vi "Calculate sensor threshold.vi"(0 "设置的起搏幅度":dbl=4.0, 5 "设定脉宽":dbl, 7 "Test Result":waveform(dbl), 9 "波形图":waveform(dbl)[](array[waveform])=[{"t0"=timestamp(3440194019.9959836 s since 1904-01-01), "dt"=1.9999999999999944e-06, "Y"=array[49999 elements], "attributes"=variant("NI_ChannelName"=variant(string "6259A/ai15"), "NI_UnitDescription"=variant(string "Volts"))}, {"t0"=timestamp(3440194019.9959836 s since 1904-01-01), "dt"=1.9999999999999944e-06, "Y"=array[49999 elements], "attributes"=variant("NI_ChannelName"=variant(string "6259A/ai21"), "NI_UnitDescription"=variant(string "Volts"))}]) -> (2 "LE":dbl, 3 "TE":dbl, 4 "VP max":dbl, 6 "VP （200u（起搏幅度））":dbl, 8 "pluse width":dbl, 10 "Vpgb（起搏幅度） 国标1":dbl, 11 "Waveform Graph Cal":waveform(dbl)(graph), 12 "VP/vh":dbl, 14 "Vpgb/vh":dbl, 15 "PW":dbl)   [LabVIEW 2016]
panel:
  out "b":dbl
  out "k":dbl
  out "element":dbl
  out "dt":dbl
  out "Waveform Graph":waveform(dbl)(graph)
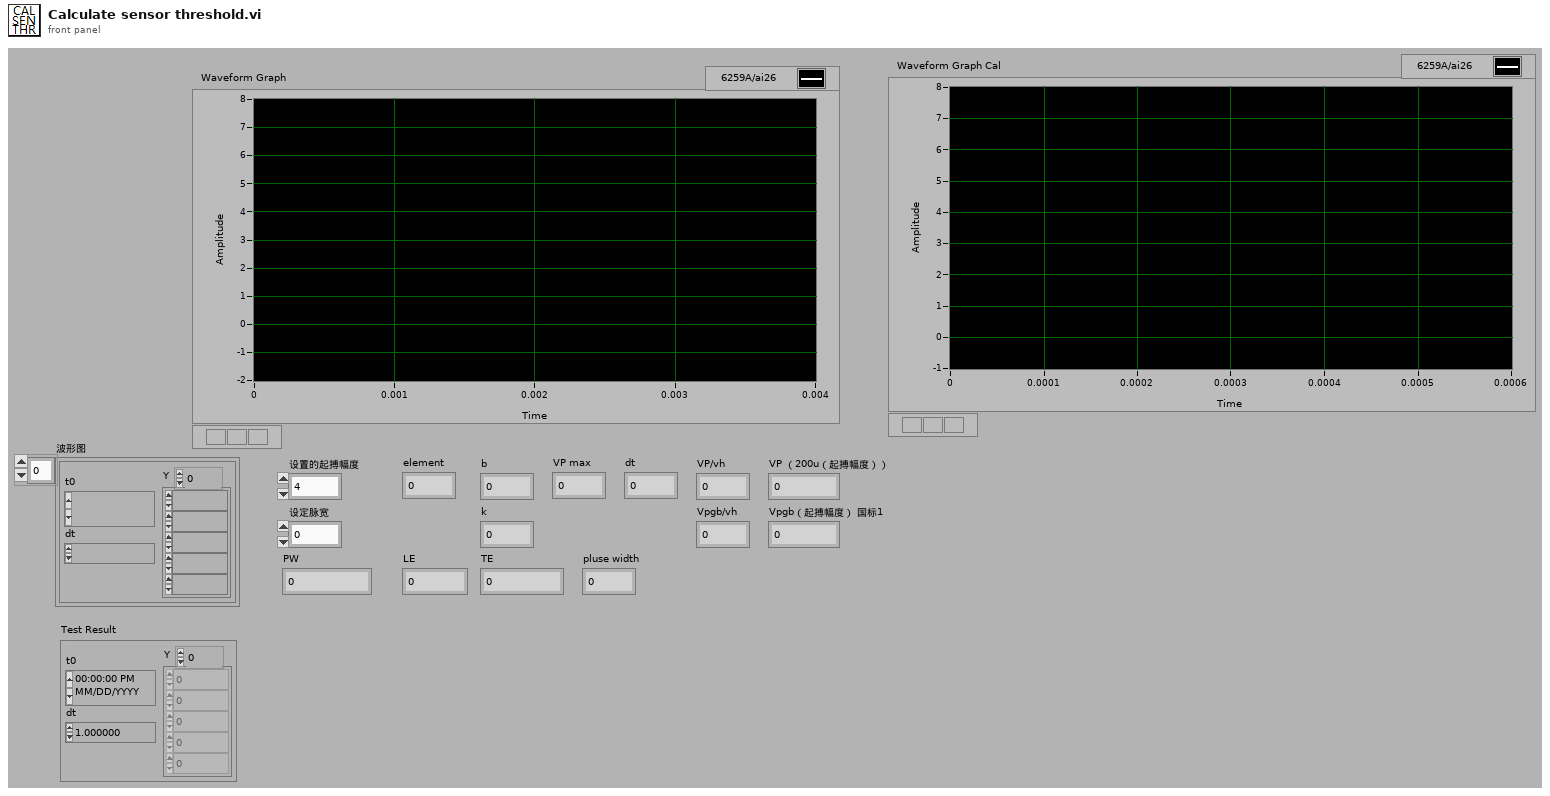
[diagram p1: front panel]
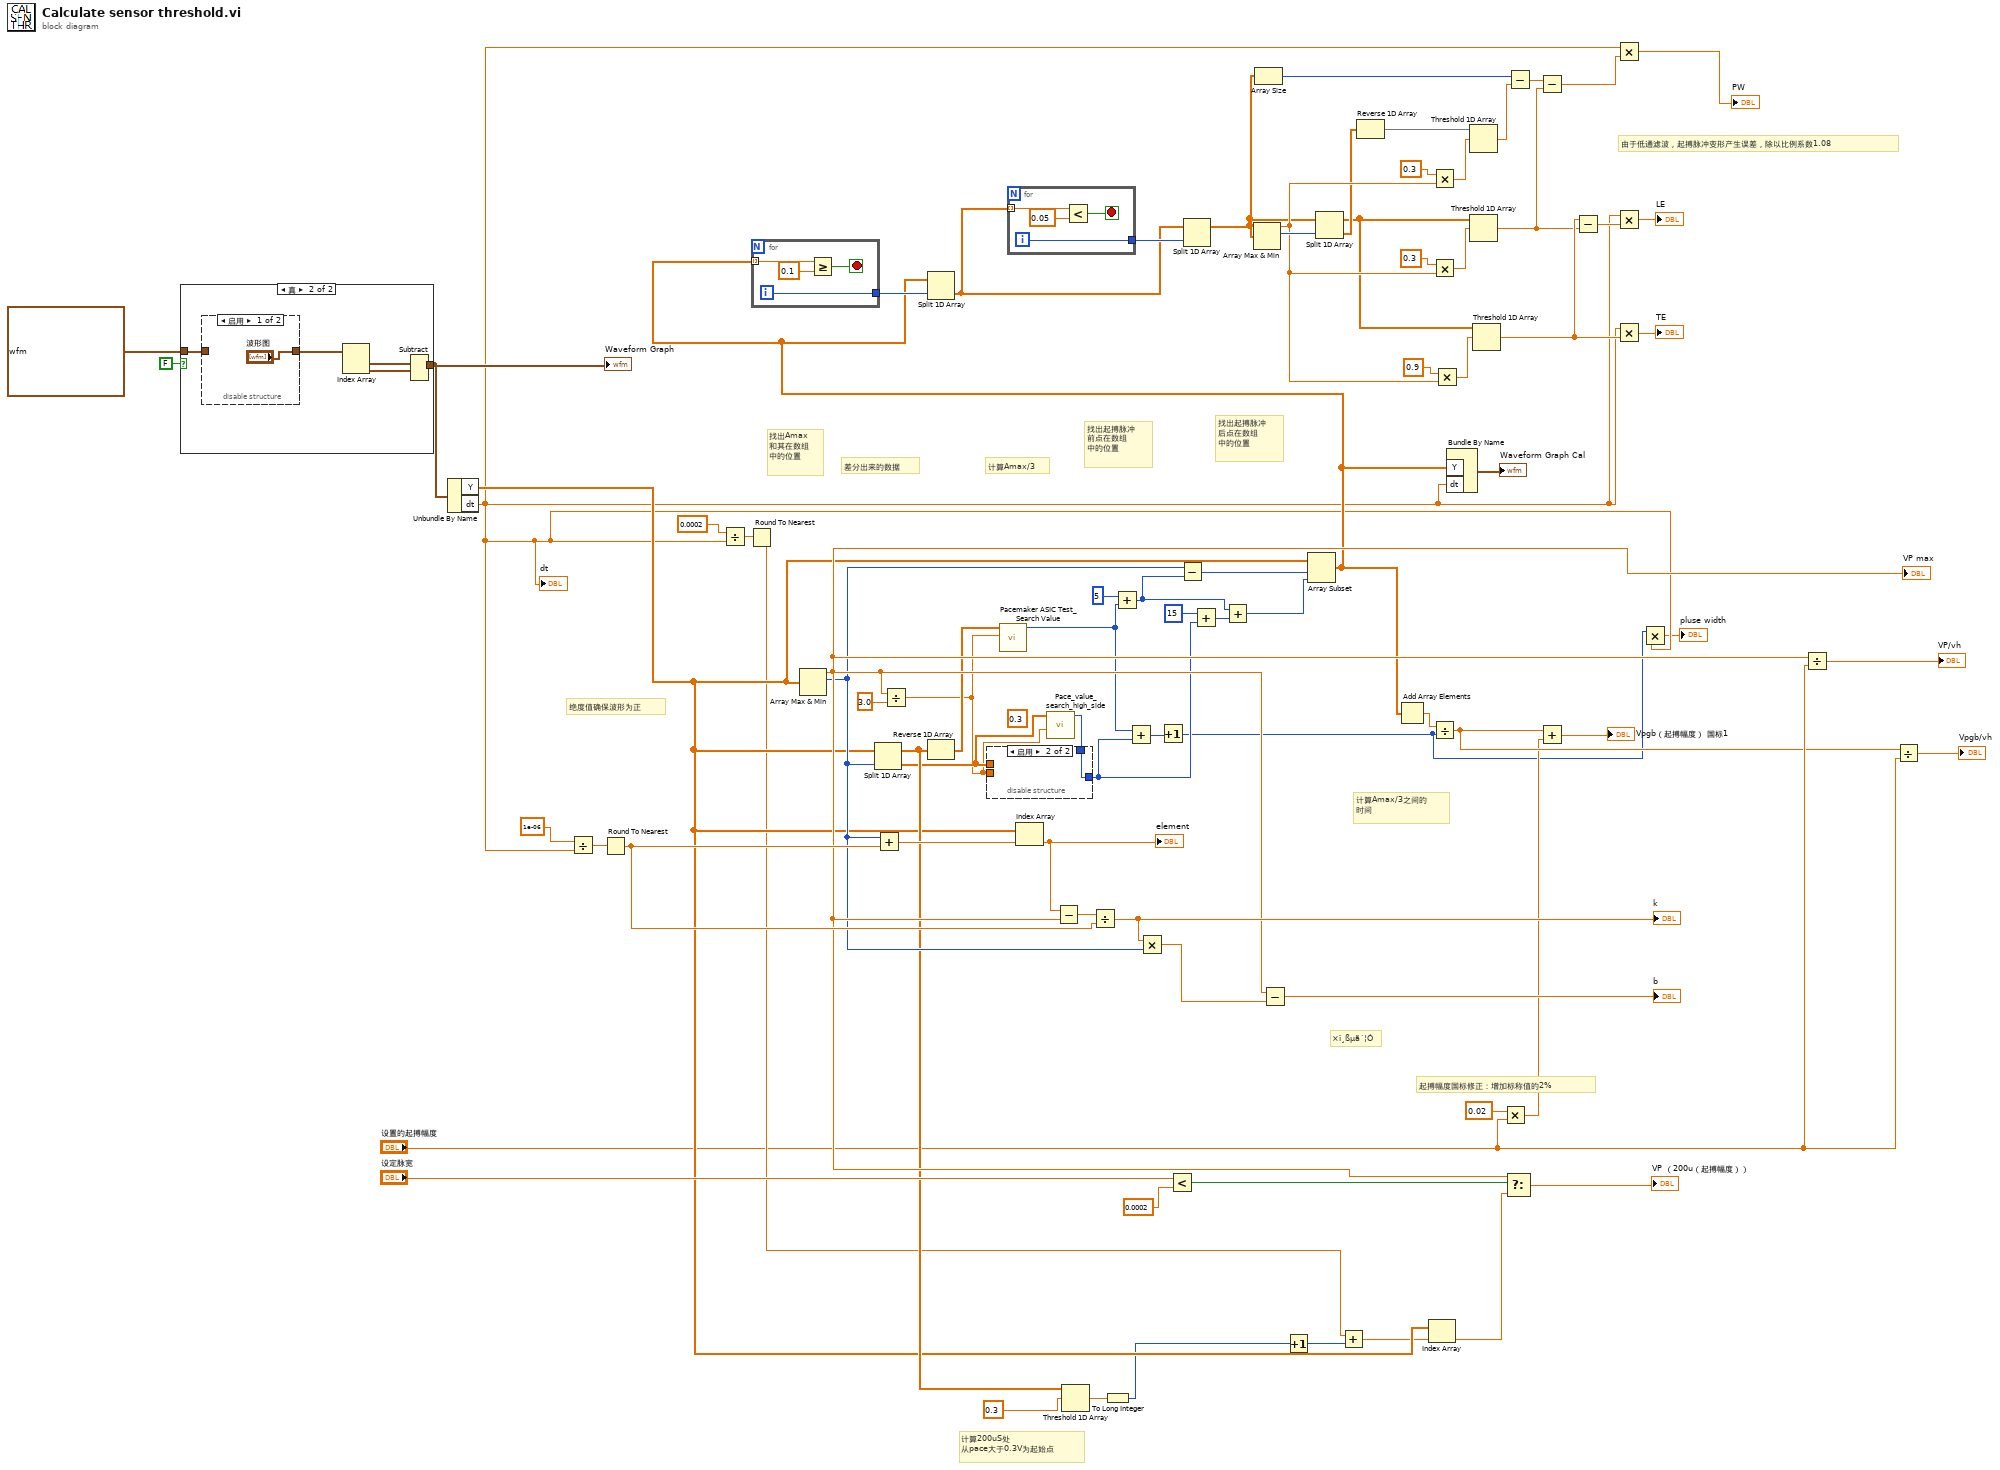
[diagram p0: block diagram]
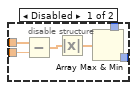
[diagram p2: hidden frame]
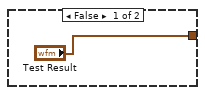
[diagram p3: hidden frame]
diagram:
  (unwired) 0.3 ("过阈值的y")
  # "起搏幅度国标修正：增加标称值的2%"
  # "由于低通滤波，起搏脉冲变形产生误差，除以比例系数1.08"
  # "找出起搏脉冲\n后点在数组\n中的位置"
  # "找出起搏脉冲\n前点在数组\n中的位置"
  # "计算Amax/3之间的\n时间"
  # "计算Amax/3"
  # "找出Amax\n和其在数组\n中的位置"
  # "×î¸ßµã´¦Ó"
  # "绝度值确保波形为正"
  # "计算200uS处\n从pace大于0.3V为起始点"
  # "差分出来的数据"
  n1 = case shown="真" FALSE {
    tunnel: waveform(dbl)[] [{"t0"=timestamp(3440384625.714352 s since 1904-01-01), "dt"=1.9999999999999944e-06, "Y"=array[49999 elements], "attributes"=variant("NI_ChannelName"=variant(string "6259A/ai17"), "NI_UnitDescription"=variant(string "Volts"))}, {"t0"=timestamp(3440384625.714352 s since 1904-01-01), "dt"=1.9999999999999944e-06, "Y"=array[49999 elements], "attributes"=variant("NI_ChannelName"=variant(string "6259A/ai20"), "NI_UnitDescription"=variant(string "Volts"))}] ("波形图 2") -> [_ w85]
    tunnel: ["Test Result" w83] -> w63
    frame False {
    }
    frame True {
      n2 = disable-structure shown="启用" {
        disable-tunnel: ["波形图" w89] -> w86
        disable-tunnel: w85 -> [_ w89]
        frame Enabled {
        }
        frame Disabled {
        }
      }
      n3 = Index Array(array=w86) -> (element #1=w87:waveform(dbl), element #2=w84:waveform(dbl))  [unwired: 2 in]
      n4 = Subtract(1:w84, 2:w87) -> (0:w83:waveform(dbl))  [unwired: 1 in, 1 out]
    }
  }
  "Waveform Graph" <- w63
  n5 = Unbundle By Name(w63) -> ("Y"=w26:dbl[], "dt"=w2:dbl)
  "dt" <- w2
  n6 = Divide(x=1e-06 ("dt 2"), y=w2) -> (x/y=w76:dbl)
  n7 = Round To Nearest(number=w76) -> (nearest integer value=w58:dbl)
  n8 = Divide(x=0.0002 ("dt 2"), y=w2) -> (x/y=w80:dbl)
  n9 = Round To Nearest(number=w80) -> (nearest integer value=w15:dbl)
  n10 = Array Max & Min(array=w26) -> (max value=w57:dbl, max index (indices)=w32:i32)  [unwired: 2 out]
  "VP max" <- w57
  n11 = Split 1D Array(array=w26, index=w32) -> (first subarray=w31:dbl[], second subarray=w6:dbl[])
  n12 = Add(x=w32, y=w58) -> (x+y=w74:dbl)
  n13 = Divide(x=w57, y=3.0) -> (x/y=w5:dbl)
  n14 = Reverse 1D Array(array=w31) -> (reversed array=w21:dbl[])
  n15 = call "Pacemaker ASIC Test_Search Value.vi"("y"=w5, "data"=w21) -> ("x"=w19:i32)  [unwired: 9 in]
  n16 = Index Array(array=w26, index=w74) -> (element=w66:dbl)
  "element" <- w66
  n17 = call "Pace_value_search_high_side.vi"("y"=w5, "data"=w6) -> ("x"=w4:i32)  [unwired: 9 in]
  n18 = disable-structure shown="启用" {
    disable-tunnel: w6 -> [w94 _]
    disable-tunnel: w5 -> [w93 _]
    disable-tunnel: [w92 w95] -> w18
    disable-tunnel: w4 -> [_ w95]
    frame Disabled {
      n19 = Subtract(x=w94, y=w93) -> (x-y=w91:dbl[])
      n20 = Absolute Value(x=w91) -> (abs(x)=w90:dbl[])
      n21 = Array Max & Min(array=w90) -> (min index (indices)=w92:i32)  [unwired: 3 out]
    }
    frame Enabled {
    }
  }
  n22 = Subtract(x=w66, y=w57) -> (x-y=w73:dbl)
  n23 = Threshold 1D Array(2:0.3 ("y"), 3:w31) -> (0:w61:dbl)  [unwired: 1 in]
  n24 = Divide(x=w73, y=w58) -> (x/y=w71:dbl)
  "k" <- w71
  n25 = To Long Integer(number=w61) -> (32bit integer=w17:i32)
  n26 = Add(x=5, y=w19) -> (x+y=w29:i32)
  n27 = Add(x=w19, y=w18) -> (x+y=w20:i32)
  n28 = Multiply(x=w71, y=w32) -> (x*y=w72:dbl)
  n29 = Increment(x=w20) -> (x+1=w3:i32)
  n30 = Less?(x="设定脉宽", y=0.0002 ("dt 2")) -> (x < y?=w67:bool)
  n31 = Subtract(x=w32, y=w29) -> (x-y=w30:i32)
  n32 = Add(x=15, y=w18) -> (x+y=w28:i32)
  n33 = Add(x=w29, y=w28) -> (x+y=w27:i32)
  n34 = Subtract(x=w57, y=w72) -> (x-y=→"b":dbl)
  n35 = Increment(x=w17) -> (x+1=w16:i32)
  n36 = Array Subset(array=w26, index=w30, length=w27) -> (w13:dbl[])
  n37 = for {
    tunnel: w13 -> [w99] mode=indexing
    tunnel: [w96] -> w56
    i -> [w96]
    stop <- w97 stop-if-true
    n38 = Greater Or Equal?(x=w99, y=0.1) -> (x >= y?=w97:bool)
  }
  n39 = Split 1D Array(array=w13, index=w56) -> (second subarray=w54:dbl[])  [unwired: 1 out]
  n40 = for {
    tunnel: w54 -> [w103] mode=indexing
    tunnel: [w100] -> w55
    i -> [w100]
    stop <- w101 stop-if-true
    n41 = Less?(x=w103, y=0.05) -> (x < y?=w101:bool)
  }
  n42 = Split 1D Array(array=w54, index=w55) -> (first subarray=w36:dbl[])  [unwired: 1 out]
  n43 = Array Max & Min(array=w36) -> (max value=w37:dbl, max index (indices)=w44:i32)  [unwired: 2 out]
  n44 = Array Size(array=w36) -> (size(s)=w49:i32)
  n45 = Split 1D Array(array=w36, index=w44) -> (first subarray=w34:dbl[], second subarray=w35:dbl[])
  n46 = Add(x=w15, y=w16) -> (x+y=w14:dbl)
  n47 = Reverse 1D Array(array=w35) -> (reversed array=w40:dbl[])
  n48 = Add Array Elements(numeric array=w13) -> (sum=w65:dbl)
  n49 = Index Array(array=w26, index=w14) -> (element=w59:dbl)
  n50 = Multiply(x=0.3, y=w37) -> (x*y=w41:dbl)
  n51 = Multiply(x=0.3, y=w37) -> (x*y=w52:dbl)
  n52 = Divide(x=w65, y=w3) -> (x/y=w10:dbl)
  n53 = Multiply(x=0.9, y=w37) -> (x*y=w50:dbl)
  n54 = Bundle By Name("Y"=w13, "dt"=w2) -> (→"Waveform Graph Cal":waveform(dbl))  [unwired: 1 in]
  n55 = Threshold 1D Array(2:w41, 3:w40) -> (0:w39:dbl)  [unwired: 1 in]
  n56 = Threshold 1D Array(2:w52, 3:w34) -> (0:w38:dbl)  [unwired: 1 in]
  n57 = Threshold 1D Array(2:w50, 3:w34) -> (0:w43:dbl)  [unwired: 1 in]
  n58 = Multiply(x=0.02, y="设置的起搏幅度") -> (x*y=w9:dbl)
  n59 = Select(t=w57, s=w67, f=w59) -> (s? t:f=→"VP （200u（起搏幅度））":dbl)
  n60 = Subtract(x=w49, y=w39) -> (x-y=w48:dbl)
  n61 = Subtract(x=w48, y=w38) -> (x-y=w23:dbl)
  n62 = Add(x=w10, y=w9) -> (x+y=→"Vpgb（起搏幅度） 国标1":dbl)
  n63 = Subtract(x=w43, y=w38) -> (x-y=w45:dbl)
  n64 = Multiply(x=w2, y=w23) -> (x*y=→"PW":dbl)
  n65 = Multiply(x=w2, y=w45) -> (x*y=→"LE":dbl)
  n66 = Multiply(x=w2, y=w43) -> (x*y=→"TE":dbl)
  n67 = Multiply(x=w3, y=w2) -> (x*y=→"pluse width":dbl)
  n68 = Divide(x=w57, y="设置的起搏幅度") -> (x/y=→"VP/vh":dbl)
  n69 = Divide(x=w10, y="设置的起搏幅度") -> (x/y=→"Vpgb/vh":dbl)
